vi "Phasor Compute Barycenter & Inertial Axes.vi"(8 "Error In":errorcluster, 11 "Phasors":csg[](array[numeric])) -> (0 "Error Out":errorcluster, 1 "Minor Axis":cluster{"x":dbl, "y":dbl}, 2 "Major Axis":cluster{"x":dbl, "y":dbl}, 3 "Barycenter":cluster{"x":sgl, "y":sgl}, 4 "Message":string)   [LabVIEW 2021, in "Phasor.lvlib"]
uses:
  Phasor.lvlib
  <vilib>/Analysis/Matrix/Datatypes/RealMatrix.ctl
  <vilib>/Analysis/7linalg.llb/SVD Option.ctl
  <vilib>/Analysis/7linalg.llb/Real SVD Decomposition.vi
  <userlib>/_OpenG.lib/array/array.llb/Filter 1D Array (CSG)__ogtk.vi
  <vilib>/Analysis/Matrix/NI_Matrix.lvlib
  <vilib>/Analysis/NI_AALPro.lvlib
  <userlib>/_OpenG.lib/array/array.llb/openg_array.lvlib
  8e8409f0-60c2-499d-bd16-3870bd156ee3.vi
panel:
  out "Valid Axes":bool
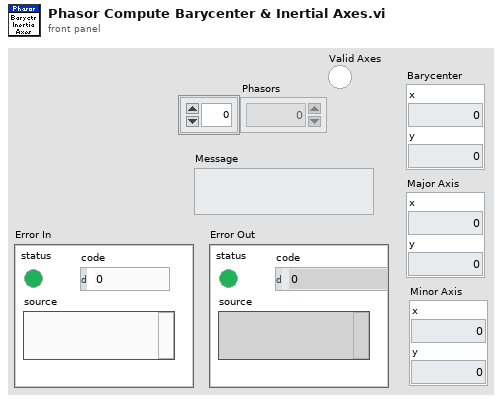
[diagram p1: front panel]
types:
  T1 = typedef "NI_Matrix.lvlib/RealMatrix.ctl" = dbl[][]
  T2 = typedef "NI_AALPro.lvlib/SVD Option.ctl" = u16
  T3 = cluster{"Real Matrix Element":dbl, "Real Matrix Element":dbl}
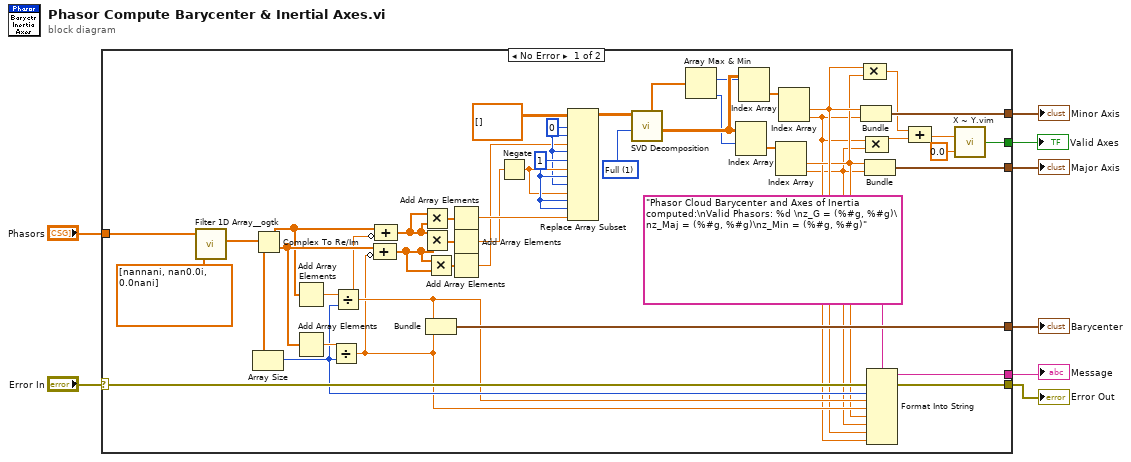
[diagram p0: block diagram]
diagram:
  n1 = case shown="No Error" "Error In" {
    selector: "Error In" -> [w24 w55]
    tunnel: "Phasors" -> [w54 _]
    tunnel: [w53 _] -> w7
    tunnel: [w49 _] -> w6
    tunnel: [w25 _] -> w5
    tunnel: [w23 _] -> w4
    tunnel: [w22 w55] -> w2
    tunnel: [w9 _] -> w1
    frame No Error {
      w38 = T2 1 items=["Thin", "Full"] ("SVD option")
      w33 = 1 ("disabled index (col)")
      w31 = 0 ("disabled index (row)")
      n2 = call-poly <userlib>:"Filter 1D Array__ogtk.vi"("items to filter"=csg[] [nan+nani, nan+0.0i, 0.0+nani] ("Element(s) to Remove"), "array"=w54) -> ("filtered array"=w42:csg[])  [unwired: 4 in, 1 out]
      n3 = Array Size(array=w42) -> (size(s)=w20:i32)
      n4 = Complex To Re/Im(x + iy=w42) -> (x=w46:sgl[], y=w47:sgl[])
      n5 = Add Array Elements(numeric array=w46) -> (sum=w39:sgl)
      n6 = Add Array Elements(numeric array=w47) -> (sum=w40:sgl)
      n7 = Divide(x=w40, y=w20) -> (x/y=w18:sgl)
      n8 = Divide(x=w39, y=w20) -> (x/y=w19:sgl)
      n9 = Compound Arithmetic op=ADD(w47, invert w18) -> (w45:sgl[])
      n10 = Compound Arithmetic op=ADD(w46, invert w19) -> (w44:sgl[])
      n11 = Multiply(x=w44, y=w44) -> (x*y=w28:sgl[])
      n12 = Multiply(x=w44, y=w45) -> (x*y=w26:sgl[])
      n13 = Multiply(x=w45, y=w45) -> (x*y=w27:sgl[])
      n14 = Bundle(w19, w18) -> (w53:cluster{sgl, sgl})  [unwired: 1 in]
      n15 = Add Array Elements(numeric array=w28) -> (sum=w34:sgl)
      n16 = Add Array Elements(numeric array=w26) -> (sum=w30:sgl)
      n17 = Add Array Elements(numeric array=w27) -> (sum=w29:sgl)
      n18 = Negate(x=w30) -> (-x=w32:sgl)
      n19 = Replace Array Subset(array=T1 [] ("matrix"), new element #1=w29, index (row) #1=w31, index (col) #1=w31, new element #2=w32, index (row) #2=w31, index (col) #2=w33, new element #3=w32, index (row) #3=w33, index (col) #3=w31, new element #4=w34, index (row) #4=w33, index (col) #4=w33) -> (w37:T1)
      n20 = call-poly <vilib>:"SVD Decomposition.vi"("SVD option"=w38, "A"=w37) -> ("Matrix V"=w52:T1, "Vector S"=w43:dbl[])  [unwired: 5 in, 3 out]
      n21 = Array Max & Min(array=w43) -> (max index (indices)=w51:i32, min index (indices)=w48:i32)  [unwired: 2 out]
      n22 = Index Array(array=w52, index (row)=w48) -> (element=w41:dbl[])  [unwired: 1 in]
      n23 = Index Array(array=w52, index (row)=w51) -> (element=w50:dbl[])  [unwired: 1 in]
      n24 = Index Array(array=w41) -> (element #1=w16:dbl, element #2=w14:dbl)  [unwired: 2 in]
      n25 = Index Array(array=w50) -> (element #1=w17:dbl, element #2=w15:dbl)  [unwired: 2 in]
      n26 = Bundle("Real Matrix Element"=w17, "Real Matrix Element"=w15) -> (w25:T3)  [unwired: 1 in]
      n27 = Compound Arithmetic op=MULTIPLY(w17, w16) -> (w12:dbl)
      n28 = Bundle("Real Matrix Element"=w16, "Real Matrix Element"=w14) -> (w49:T3)  [unwired: 1 in]
      n29 = Compound Arithmetic op=MULTIPLY(w15, w14) -> (w13:dbl)
      n30 = Format Into String(format string="Phasor Cloud Barycenter and Axes of Inertia computed:\nValid Phasors: %d \nz_G = (%#g, %#g)\nz_Maj = (%#g, %#g)\nz_Min = (%#g, %#g)", error in=w24, w20, w19, w18, w16, w14, w17, w15) -> (resulting string=w23:string, error out=w22:errorcluster)  [unwired: 1 in]
      n31 = Compound Arithmetic op=ADD(w12, w13) -> (w11:dbl)
      n32 = call "X ~ Y.vim"("X"=w11, "Y"=0.0) -> ("X ~= Y?"=w9:bool)  [unwired: 13 in]
    }
    frame Error {
    }
  }
  "Barycenter" <- w7
  "Major Axis" <- w6
  "Minor Axis" <- w5
  "Error Out" <- w2
  "Message" <- w4
  "Valid Axes" <- w1
